vi "WLAN -.Create Scriptvi.vi"(0 "Initial Delay (ms)":u32, 5 "Number of Packets":i32=50 min=1 max=1000) -> (4 "resulting script":string)   [LabVIEW 2011]
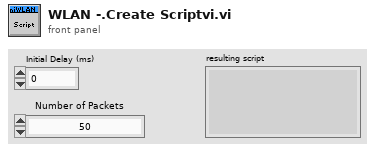
[diagram p1: front panel]
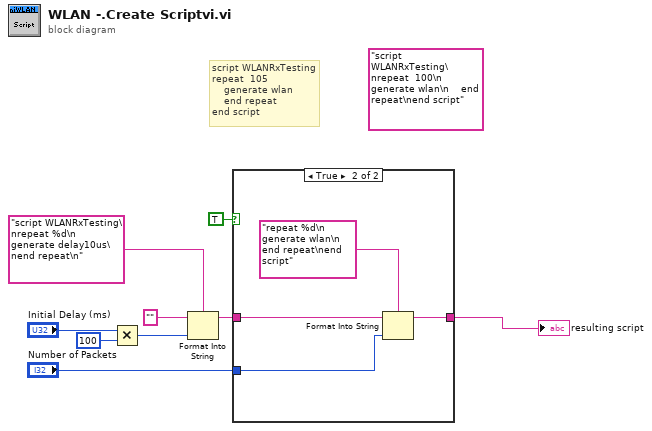
[diagram p0: block diagram]
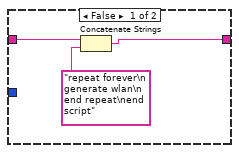
[diagram p2: hidden frame]
diagram:
  (unwired) "script WLANRxTesting\nrepeat  100\n    generate wlan\n    end repeat\nend script" ("Script")
  # "script WLANRxTesting\nrepeat  105\n    generate wlan\n    end repeat\nend script"
  n1 = Multiply(x="Initial Delay (ms)", y=u32 100) -> (x*y=w3:u32)
  n2 = Format Into String(format string="script WLANRxTesting\nrepeat %d\n    generate delay10us\nend repeat\n" ("Script"), initial string="", w3) -> (resulting string=w7:string)  [unwired: 1 in, 1 out]
  n3 = case shown="True" TRUE {
    tunnel: w7 -> [w12 w16]
    tunnel: "Number of Packets" -> [_ w15]
    tunnel: [w10 w13] -> w1
    frame False {
      n4 = Concatenate Strings(w12, "repeat forever\n    generate wlan\n    end repeat\nend script" ("Script")) -> (w10:string)
    }
    frame True {
      n5 = Format Into String(format string="repeat %d\n    generate wlan\n    end repeat\nend script" ("Script"), initial string=w16, w15) -> (resulting string=w13:string)  [unwired: 1 in, 1 out]
    }
  }
  "resulting script" <- w1
